vi "status code.vi"(0 "status code":string) -> (1 "Relay 24-31":bool[](array[boolean]), 2 "Relay 16-23":bool[](array[boolean]), 3 "Relay 8-15":bool[](array[boolean]), 4 "Relay 0-7":bool[](array[boolean]))   [LabVIEW 2016]
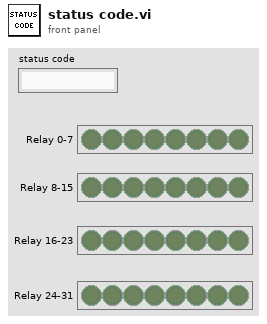
[diagram p1: front panel]
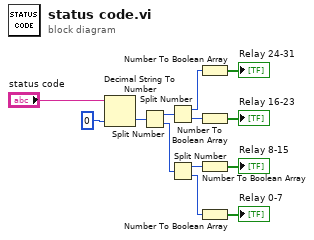
[diagram p0: block diagram]
diagram:
  n1 = Decimal String To Number(string="status code", default (0L)=u32 0 ("default (0 I32)")) -> (number=w11:u32)  [unwired: 1 in, 1 out]
  n2 = Split Number(x=w11) -> (hi(x)=w10:u16, lo(x)=w9:u16)
  n3 = Split Number(x=w10) -> (hi(x)=w5:u8, lo(x)=w4:u8)
  n4 = Split Number(x=w9) -> (hi(x)=w6:u8, lo(x)=w8:u8)
  n5 = Number To Boolean Array(number=w5) -> (Boolean array=→"Relay 24-31":bool[])
  n6 = Number To Boolean Array(number=w4) -> (Boolean array=→"Relay 16-23":bool[])
  n7 = Number To Boolean Array(number=w6) -> (Boolean array=→"Relay 8-15":bool[])
  n8 = Number To Boolean Array(number=w8) -> (Boolean array=→"Relay 0-7":bool[])
